vi "Analyze_IV.vi"(8 "Diff bin size":dbl, 9 "Points to chop off the bottom edge":i32, 10 "Points to chop off the top edge":i32, 11 "A vs B IN":cluster{dbl[], dbl[]}[](array[cluster])) -> (0 "dI/dV values":dbl[](graph), 1 "Vsrc values":dbl[](graph), 2 "dI/dV curve subsection":cluster{dbl[], dbl[]}(graph), 3 "IV curve subsection":cluster{dbl[], dbl[]}(graph))   [LabVIEW 2016]
panel:
  out "min index(es)":i32
  out "max index(es)":i32
  out "Entire Current":dbl[](graph)
  out "Entire Vsrc":dbl[](graph)
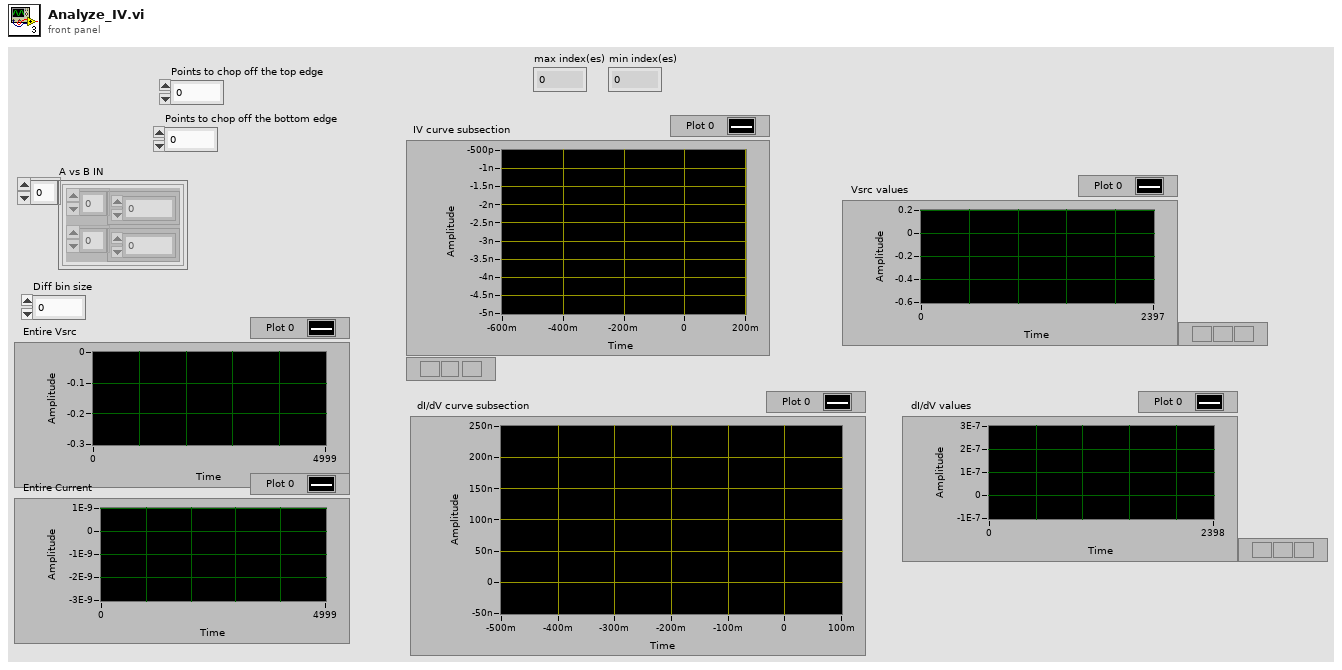
[diagram p1: front panel]
types:
  T1 = cluster{"Decimated Array":dbl[], "Decimated Array":dbl[]}
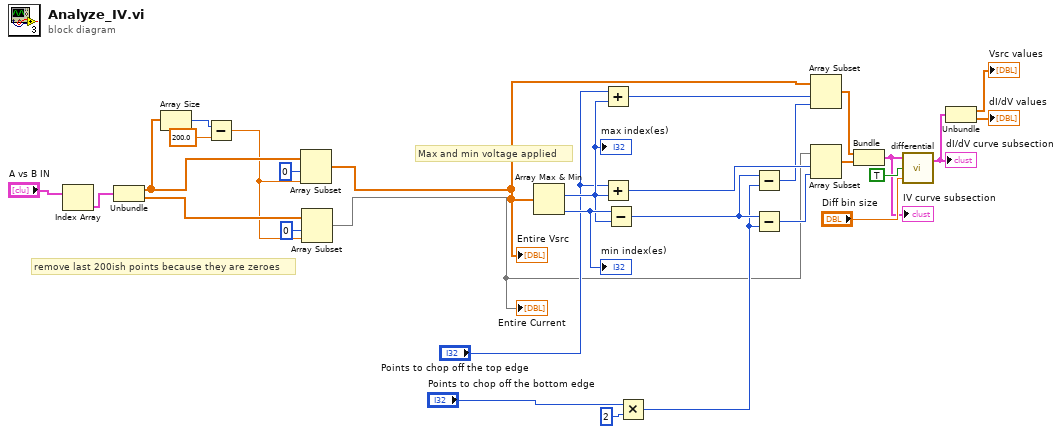
[diagram p0: block diagram]
diagram:
  # "remove last 200ish points because they are zeroes"
  # "Max and min voltage applied"
  n1 = Index Array(array="A vs B IN") -> (element=w10:cluster{dbl[], dbl[]})  [unwired: 1 in]
  n2 = Unbundle(w10) -> (w6:dbl[], w9:dbl[])
  n3 = Array Size(array=w6) -> (size(s)=w4:i32)
  n4 = Subtract(x=w4, y=200.0) -> (x-y=w3:dbl)
  n5 = Array Subset(array=w6, index=0, length=w3) -> (w8:dbl[])
  "Entire Vsrc" <- w8
  n6 = Array Subset(array=w9, index=0, length=w3) -> (w7:dbl[])
  "Entire Current" <- w7
  n7 = Array Max & Min(array=w8) -> (max index (indices)=w20:i32, min index (indices)=w27:i32)  [unwired: 2 out]
  "max index(es)" <- w20
  "min index(es)" <- w27
  n8 = Add(x="Points to chop off the top edge", y=w20) -> (x+y=w24:i32)
  n9 = Add(x="Points to chop off the top edge", y=w20) -> (x+y=w23:i32)
  n10 = Subtract(x=w27, y=w20) -> (x-y=w19:i32)
  n11 = Multiply(x="Points to chop off the bottom edge", y=2) -> (x*y=w15:i32)
  n12 = Subtract(x=w19, y=w15) -> (x-y=w22:i32)
  n13 = Subtract(x=w19, y=w15) -> (x-y=w21:i32)
  n14 = Array Subset(array=w8, index=w24, length=w22) -> (w14:dbl[])
  n15 = Array Subset(array=w7, index=w23, length=w21) -> (w13:dbl[])
  n16 = Bundle(w14, w13) -> (w26:cluster{dbl[], dbl[]})  [unwired: 1 in]
  "IV curve subsection" <- w26
  n17 = call <userlib>:"differential.vi"("Numeric"="Diff bin size", "dy/dx vs x"=TRUE, "A vs B 2"=w26) -> ("A vs B 3"=w25:T1)  [unwired: 1 in]
  "dI/dV curve subsection" <- w25
  n18 = Unbundle(w25) -> ("Decimated Array"=→"Vsrc values":dbl[], "Decimated Array"=→"dI/dV values":dbl[])
